vi "Apply Ref Plane Extension.vi"(0 "Sxx Data":cdb[](array[numeric]), 5 "Frequencies":dbl[](array[numeric]), 7 "Ref Plane Extension Time":dbl, 11 "Error In":errorcluster) -> (4 "Sxx Data - Ref Plane Shifted":cdb[](array[numeric]), 15 "Error Out":errorcluster)   [LabVIEW 2013]
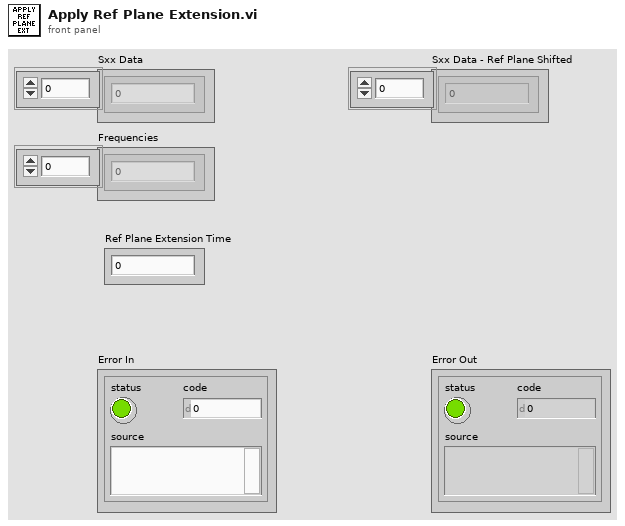
[diagram p1: front panel]
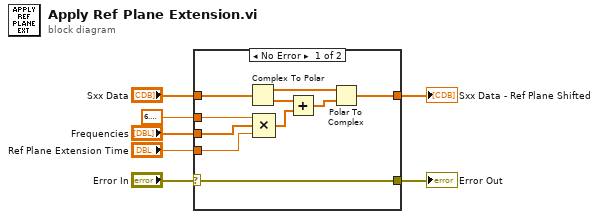
[diagram p0: block diagram]
diagram:
  n1 = case shown="No Error" "Error In" {
    selector: "Error In" -> [w17 w18]
    tunnel: "Sxx Data" -> [w10 w19]
    tunnel: [w9 w19] -> w6
    tunnel: [w17 w18] -> w4
    tunnel: "Frequencies" -> [w13 _]
    tunnel: "Ref Plane Extension Time" -> [w12 _]
    tunnel: 6.283185307179586 -> [w11 _]
    frame No Error {
      n2 = Complex To Polar(r * e^(i*theta)=w10) -> (r=w14:dbl[], theta=w15:dbl[])
      n3 = Compound Arithmetic op=MULTIPLY(w11, w13, w12) -> (w16:dbl[])
      n4 = Add(x=w15, y=w16) -> (x+y=w8:dbl[])
      n5 = Polar To Complex(1:w8, 2:w14) -> (0:w9:cdb[])
    }
    frame Error {
    }
  }
  "Sxx Data - Ref Plane Shifted" <- w6
  "Error Out" <- w4
